vi "快捷购买信息.vi"() -> ()   [LabVIEW 2020]
panel:
  out "地址：":string
  out "电话：":string
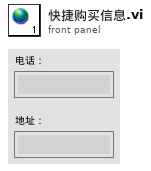
[diagram p1: front panel]
diagram:
